vi "Write Data to 128-bit FIFO.vi"(7 "FIFO In":refnum<k21>="ContinuousInputStream", 9 "Input Valid":bool, 11 "Data":i16[](array[numeric])=[0, 0, 0, 0, 0, 0, 0, 0]) -> (0 "FIFO Timed Out?":bool, 1 "Ever Timed Out?":bool)   [LabVIEW 2011]
uses:
  <vilib>/rvi/DataTransferAndStorage/Container/Common/niFpgaContainerExecOnDevCompGetState.vi
  <vilib>/rvi/FIFO/Fifo_Resource/nirvififoEmulationSetSize.vi
  <vilib>/rvi/DataTransferAndStorage/Container/Common/niFpgaContainerGetUniqueNameForEmu.vi
  <vilib>/rvi/interface/RandomDataEmulation/nirviRandomDataFPGAFIFO.vi
  <vilib>/rvi/interface/RandomDataEmulation/niFpgaRandomDataHandleErrors.vi
  <vilib>/rvi/eio/common/nirviEmuReportErrorAndStop.vi
  <vilib>/rvi/DataTransferAndStorage/Container/XNode/niFpgaContainer.xnode
  <vilib>/rvi/FIFO/Fifo_Resource/niFpgaFifoEmulationRefIn.vi
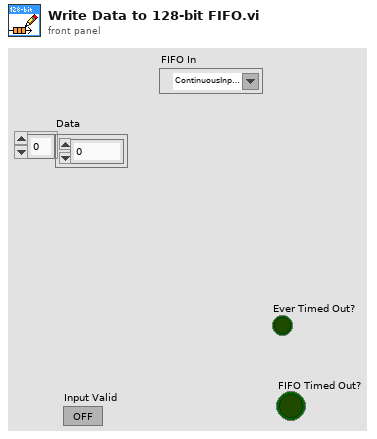
[diagram p1: front panel]
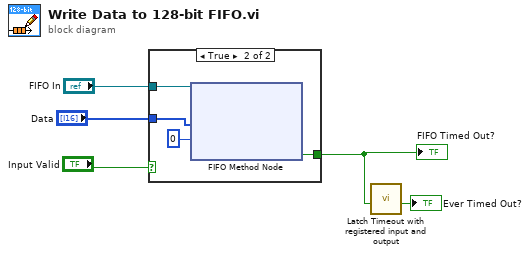
[diagram p0: block diagram]
diagram:
  n1 = case shown="True" "Input Valid" {
    tunnel: "FIFO In" -> [_ w8]
    tunnel: [_ w7] -> w2
    tunnel: "Data" -> [_ w6]
    frame False {
    }
    frame True {
      n2 = xnode ("FIFO Method Node")("Element"=w6, "Timeout"=0, "FIFO In"=w8) -> ("Timed Out?"=w7:bool)  [unwired: 1 out]
    }
  }
  "FIFO Timed Out?" <- w2
  n3 = call <userlib>:"Latch Timeout with registered input and output.vi"("Timeout?"=w2) -> ("Ever Timed Out?"=→"Ever Timed Out?":bool)  [unwired: 10 in]
